vi "Ejercicio 3.4.vi"() -> ()   [LabVIEW 2021]
uses:
  <vilib>/numeric/Random Number (Range) I64.vi
  <vilib>/numeric/sub_Random U32.vi
panel:
  out "XY Graph 2":cluster{i32[], i64[]}(graph)
  out "XY Graph 1":cluster{i32[], i64[]}(graph)
  out "Array":dbl[][](array[numeric])
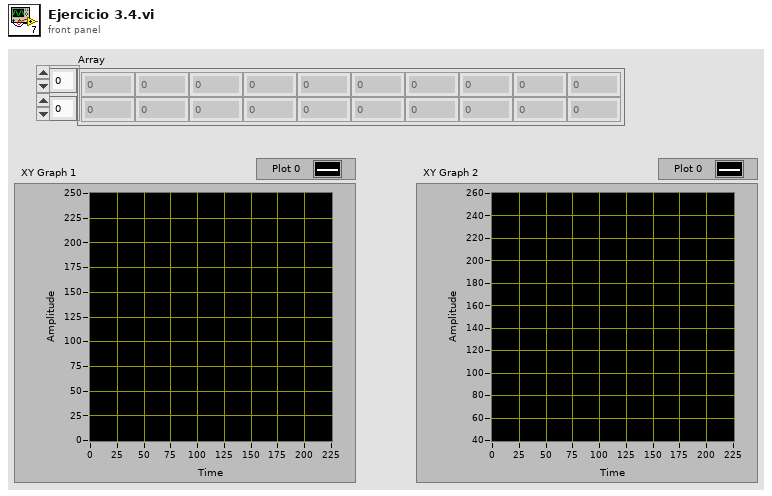
[diagram p1: front panel]
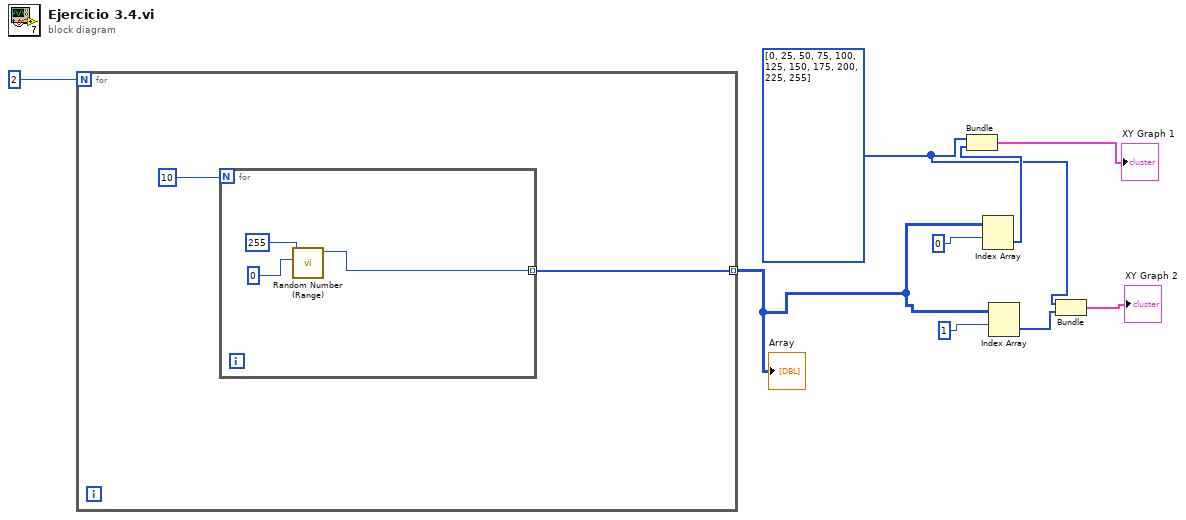
[diagram p0: block diagram]
diagram:
  w1 = i32[] [0, 25, 50, 75, 100, 125, 150, 175, 200, 225, 255]
  n1 = for {
    N: 2 -> [_]
    tunnel: [w10] -> w6 mode=indexing
    n2 = for {
      N: 10 -> [_]
      tunnel: [w14] -> w10 mode=indexing
      n3 = call-poly <vilib>:"Random Number (Range).vi"("lower bound (-100)"=0, "upper bound (100)"=255) -> ("number"=w14:i64)  [unwired: 9 in]
    }
  }
  "Array" <- w6
  n4 = Index Array(array=w6, index (row)=0) -> (element=w3:i64[])  [unwired: 1 in]
  n5 = Bundle(w1, w3) -> (→"XY Graph 1":cluster{i32[], i64[]})  [unwired: 1 in]
  n6 = Index Array(array=w6, index (row)=1) -> (element=w2:i64[])  [unwired: 1 in]
  n7 = Bundle(w1, w2) -> (→"XY Graph 2":cluster{i32[], i64[]})  [unwired: 1 in]
